vi "ASS2-Demodulating.vi"() -> ()   [LabVIEW 2018]
uses:
  <vilib>/measure/NI_MABase.lvlib
panel:
  out "Modulating signal":dynamicdata(graph)
  out "Demodulating signal":dynamicdata(graph)
  out "Modulated signal":dynamicdata(graph)
  in  "seed":i32=-1
  in  "amplitude 2":dbl=1.0 format="%.2p"
  in  "sampling info":cluster{"Fs":dbl, "#s":dbl}={"Fs"=1000.0, "#s"=1000.0} {"Fs" format="%.2p"}
  in  "amplitude":dbl=1.0 format="%0.2p"
  in  "frequency":dbl=10.0 format="%0.2p"
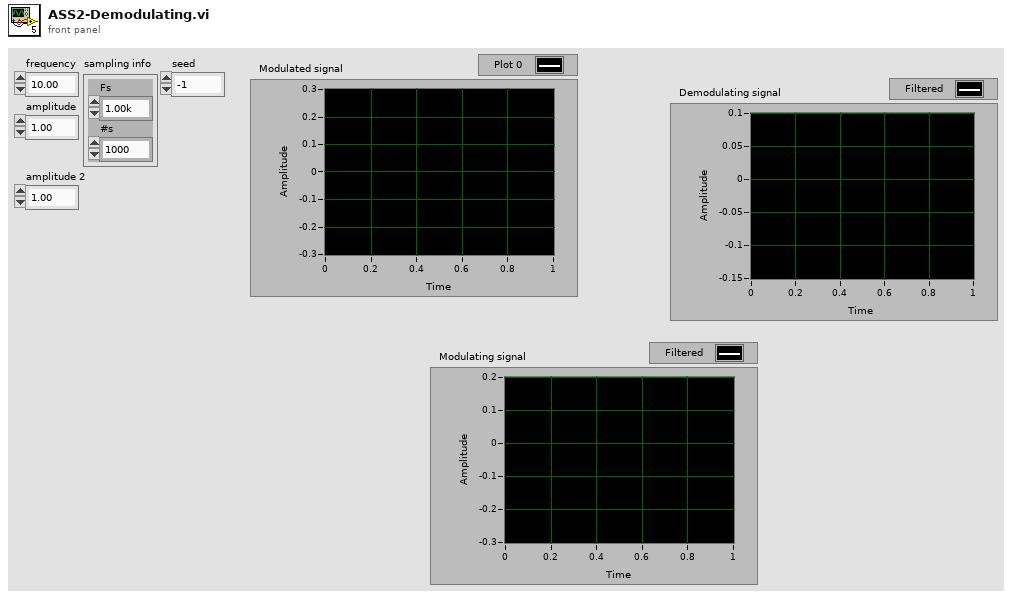
[diagram p1: front panel]
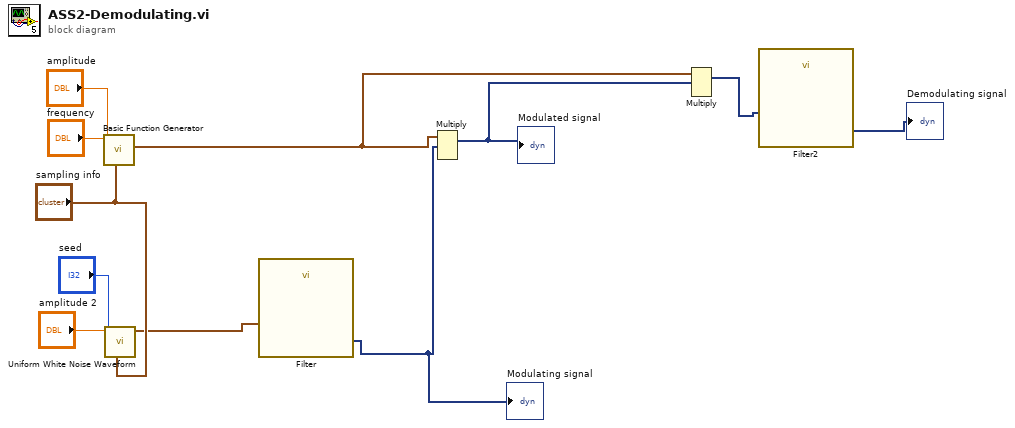
[diagram p0: block diagram]
diagram:
  n1 = call <vilib>:"Basic Function Generator.vi"("sampling info"="sampling info", "amplitude"="amplitude", "frequency"="frequency") -> ("signal out"=w5:waveform(dbl))  [unwired: 6 in, 2 out]
  n2 = call <vilib>:"Uniform White Noise Waveform.vi"("sampling info"="sampling info", "seed"="seed", "amplitude"="amplitude 2") -> ("signal out"=w6:waveform(dbl))  [unwired: 7 in, 1 out]
  n3 = call "Filter"("Signal"=w6) -> ("Filtered Signal"=w1:dynamicdata)  [unwired: 9 in, 1 out]
  "Modulating signal" <- w1
  n4 = Multiply(1:w1, 2:w5) -> (0:w4:dynamicdata)  [unwired: 1 in, 1 out]
  "Modulated signal" <- w4
  n5 = Multiply(1:w4, 2:w5) -> (0:w3:dynamicdata)  [unwired: 1 in, 1 out]
  n6 = call "Filter2"("Signal"=w3) -> ("Filtered Signal"=→"Demodulating signal":dynamicdata)  [unwired: 9 in, 1 out]
